vi "Restore Configuration.vi"(8 "error in (no error)":errorcluster, 10 "File path":path, 11 "Monitor-Pulse in":refnum<class "Monitor-Pulse.lvclass">) -> (0 "error out":errorcluster, 1 "Section out":string, 2 "File path out":path, 3 "Monitor-Pulse out":refnum<class "Monitor-Pulse.lvclass">)   [LabVIEW 2016, in "Monitor-Pulse.lvclass"]
uses:
  Monitor-Pulse.lvclass
  C:/github/Measure_core/Da Base/Da Base.lvclass
  Measure_core/Da Base/Da Base.lvclass/Da Base.ctl
  Monitor-Pulse.lvclass/Monitor-Pulse.ctl
  NHMFL_Core/Libraries/Queued Listbox/Queued Listbox.xctl
  Measure_core/da Base/Read Name.vi
  <vilib>/Utility/error.llb/Error Cluster From Error Code.vi
  <vilib>/ErrorRing/Error Ring.xnode
  Measure_core/Controllers/Application Controller/Application Controller.lvclass
  <vilib>/Utility/config.llb/NI_LVConfig.lvlib
panel:
  out "Array":string[](array[string])
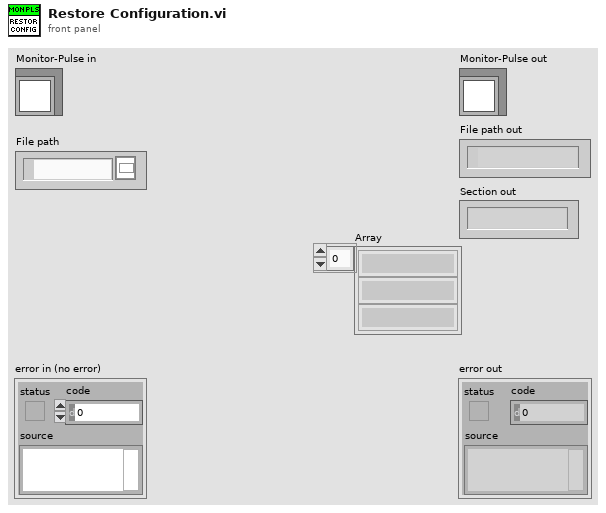
[diagram p1: front panel]
types:
  T1 = typedef "NI_LVConfig.lvlib/Config Data RefNum.ctl" = refnum<k1>
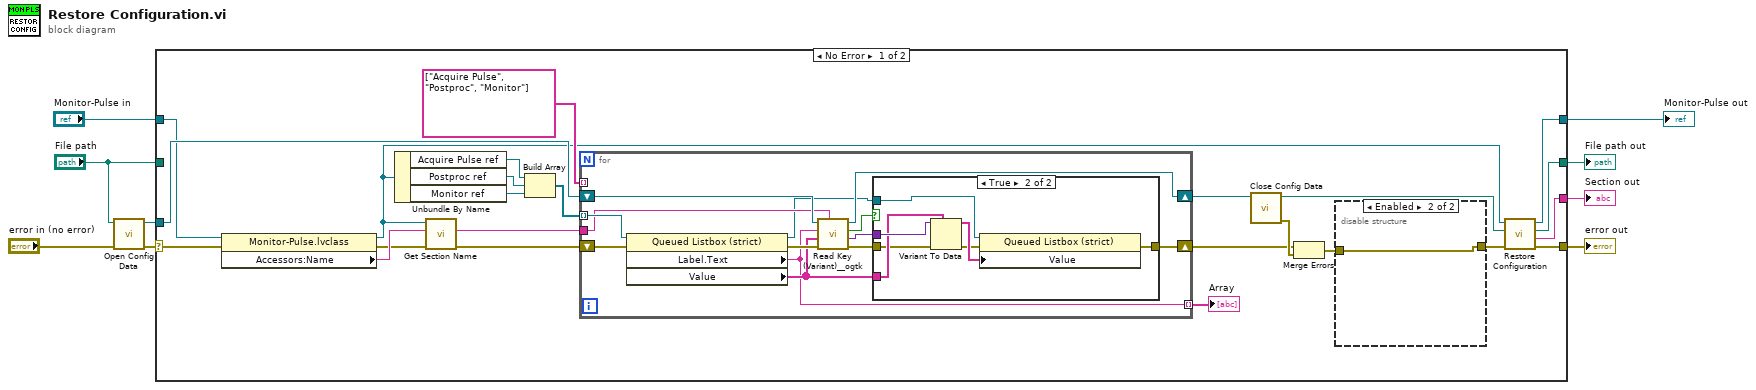
[diagram p0: block diagram]
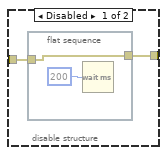
[diagram p2: hidden frame]
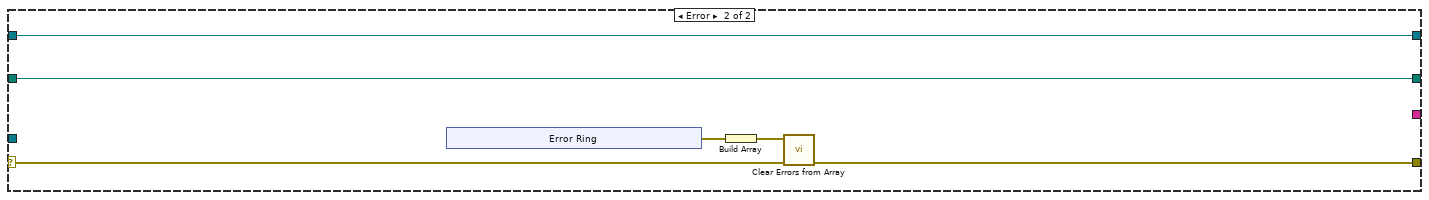
[diagram p4: hidden frame]
diagram:
  n1 = call <vilib>:"Open Config Data.vi"("error in (no error)"="error in (no error)", "configuration file path"="File path") -> ("error out"=w2:errorcluster, "refnum"=w9:T1)  [unwired: 7 in, 1 out]
  n2 = case shown="No Error" w2 {
    selector: w2 -> [w10 w61]
    tunnel: w9 -> [w29 _]
    tunnel: [w21 _] -> w8
    tunnel: [w18 w65] -> w7
    tunnel: "Monitor-Pulse in" -> [w17 w65]
    tunnel: [w16 w60] -> w5
    tunnel: [w13 w64] -> w4
    tunnel: "File path" -> [_ w64]
    frame No Error {
      n3 = property class="Monitor-Pulse.lvclass"(reference=w17, error in=w10) -> (reference out=w19:refnum<class "Monitor-Pulse.lvclass">, error out=w22:errorcluster, "Accessors:Name"=w23:string)
      n4 = Unbundle By Name(w19) -> ("Acquire Pulse ref"=w33:refnum<vi>, "Postproc ref"=w32:refnum<vi>, "Monitor ref"=w31:refnum<vi>)
      n5 = call "Get Section Name.vi"("Error In"=w22, "Object name"=w23, "object"=w19) -> ("Error Out"=w11:errorcluster, "Section out"=w20:string)  [unwired: 7 in]
      n6 = Build Array(w33, w32, w31) -> (w30:refnum<vi>[])
      n7 = for {
        tunnel: w30 -> [w51] mode=indexing
        shift-right: [w41] -> w27
        shift-left: w11 -> [w50]
        shift-right: [w48] -> w26
        shift-left: w29 -> [w49]
        tunnel: w20 -> [w46]
        tunnel: string[] ["Acquire Pulse", "Postproc", "Monitor"] -> [_] mode=indexing
        tunnel: [w40] -> w24 mode=indexing
        n8 = property class="Queued Listbox (strict)"(reference=w51, error in=w50) -> (reference out=w45:refnum<vi>, error out=w47:errorcluster, "Label.Text"=w40:string, "Value"=w43:string[])
        n9 = call <userlib>:"Read Key (Variant)__ogtk.vi"("section"=w46, "error in (no error)"=w47, "type"=w43, "key (optional)"=w40, "refnum"=w49) -> ("error out"=w42:errorcluster, "key-value"=w44:variant, "found?"=w39:bool, "refnum out"=w48:T1)  [unwired: 3 in]
        n10 = case shown="True" w39 {
          tunnel: w45 -> [_ w59]
          tunnel: w44 -> [_ w58]
          tunnel: w43 -> [_ w57]
          tunnel: w42 -> [w52 w55]
          tunnel: [w52 w53] -> w41
          frame False {
          }
          frame True {
            n11 = Variant To Data(error in=w55, type=w57, Variant=w58) -> (data=w56:string[], error out=w54:errorcluster)
            n12 = property class="Queued Listbox (strict)"(reference=w59, error in=w54, "Value"=w56) -> (error out=w53:errorcluster)  [unwired: 1 out]
          }
        }
      }
      "Array" <- w24
      n13 = call <vilib>:"Close Config Data.vi"("refnum"=w26) -> ("error out"=w28:errorcluster, "file path"=w14:path)  [unwired: 9 in]
      n14 = Merge Errors(w27, w28) -> (w15:errorcluster)
      n15 = disable-structure shown="Enabled" {
        disable-tunnel: w15 -> [w35 w38]
        disable-tunnel: [w34 w38] -> w12
        frame Disabled {
          n16 = flat-sequence {
            tunnel: w35 -> [w37]
            tunnel: [w37] -> w34
            frame #0 {
              n17 = Wait (ms)(milliseconds to wait=u32 200) -> ()  [unwired: 1 out]
            }
          }
        }
        frame Enabled {
        }
      }
      n18 = call-parent "Restore Configuration.vi"("error in (no error)"=w12, "File path"=w14, "Measure Object in"=w19) -> ("error out"=w16:errorcluster, "Section out"=w21:string, "File path out"=w13:path, "Measure Object out"=w18:refnum<class "Monitor-Pulse.lvclass">)  [unwired: 5 in]
    }
    frame Error {
      n19 = xnode "Error Ring"() -> ("error out"=w63:errorcluster)
      n20 = Build Array(w63) -> (w62:errorcluster[])
      n21 = call "Clear Errors from Array.vi"("Error In"=w61, "Errors to clear"=w62) -> ("Error Out"=w60:errorcluster)  [unwired: 8 in, 1 out]
    }
  }
  "error out" <- w5
  "Monitor-Pulse out" <- w7
  "File path out" <- w4
  "Section out" <- w8
